vi "Write rotatorTracking.vi"(8 "error in (no error)":errorcluster, 10 "RotatorTracking.lvclass":refnum<class "RotatorTracking.lvclass">, 11 "TCSMccStatus in":refnum<class "TCSMccStatus.lvclass">) -> (0 "error out":errorcluster, 3 "TCSMccStatus out":refnum<class "TCSMccStatus.lvclass">)   [LabVIEW 2014, in "TCSDataDefinitions.lvlib" / "TCSMountControlStatus.lvlib" / "TCSMccStatus.lvclass"]
uses:
  TCSMccStatus.lvclass
  RotatorTracking/RotatorTracking/RotatorTracking.lvclass
  TCSMccStatus.lvclass/TCSMccStatus.ctl
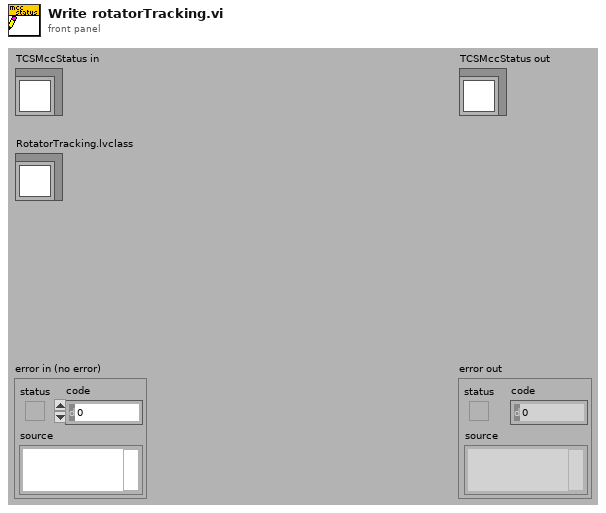
[diagram p1: front panel]
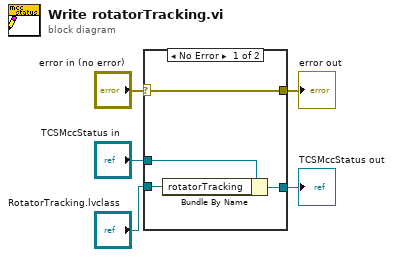
[diagram p0: block diagram]
diagram:
  n1 = case shown="No Error" "error in (no error)" {
    selector: "error in (no error)" -> [w9 w10]
    tunnel: [w9 w10] -> w4
    tunnel: [w7 w11] -> w2
    tunnel: "TCSMccStatus in" -> [w8 w11]
    tunnel: "RotatorTracking.lvclass" -> [w6 _]
    frame No Error {
      n2 = Bundle By Name(cluster=w8, "rotatorTracking"=w6) -> (w7:refnum<class "TCSMccStatus.lvclass">)
    }
    frame Error {
    }
  }
  "error out" <- w4
  "TCSMccStatus out" <- w2
